vi "PlayFile.vi"(11 "Old Files":T1[](array[typedef])) -> ()   [LabVIEW 2022 SP3]
uses:
  Curtin1_Label.ctl
panel:
  in  "Save Convolve":bool
  in  "Convolve":bool
  in  "Save Button":bool
  in  "Play Button":bool
  in  "Instruments":u16(ring) items=["JacksonStrad H.AvR"]
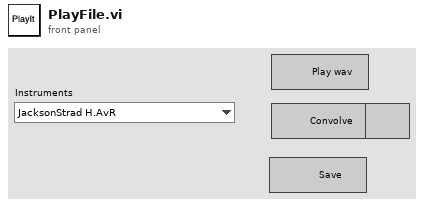
[diagram p1: front panel]
types:
  T1 = typedef "Curtin1_Label.ctl" = cluster{"Show?":bool, "Name":string, "Color":u32, "Path":path, "Show Notes":bool}
  T2 = typedef "PreferencesControl.ctl" = cluster{"Name of test":string, "Date":timestamp, "Location":string, "Template":string, "Soundcard":string, "resolution":u16, "Sampling rate":u16, "Ch1 Gain ":dbl, "Ch2 Gain":dbl, "Sample time (s)":dbl, "Pre-trigger (s)":dbl, "Hammer Threshold":dbl, "Positions":i16, "Taps/Position":i16, "Set Names":string, "Freq resolution":dbl, "Hammer cutoff":dbl, "Mic cutoff":dbl, "Double bounce ":dbl, "Hammer Cal":dbl, "dB Offset":dbl, "Accel Cal":dbl, "Vibrometer Cal":dbl, "Mic Cal":dbl, "Output":u16, "Voltage Cal":dbl, "Vibrometer Port":refnum<visa-resource-name>, "Range":u16, "High Pass":u16, "Bandwidth":u16, "X Range":cluster{"Minimum":dbl, "Maximum":dbl, "Increment":dbl, "Minor Increment":dbl, "Start":dbl}[], "Y Range":cluster{"Minimum":dbl, "Maximum":dbl, "Increment":dbl, "Minor Increment":dbl, "Start":dbl}[], "dB Spread":dbl, "Trigger":u16, "Ch_1":u8, "Ch_2":u8, "flip?":bool, "60Hz":bool, "Time offset":dbl, "Piezo Cal":dbl, "Default Notes":string}
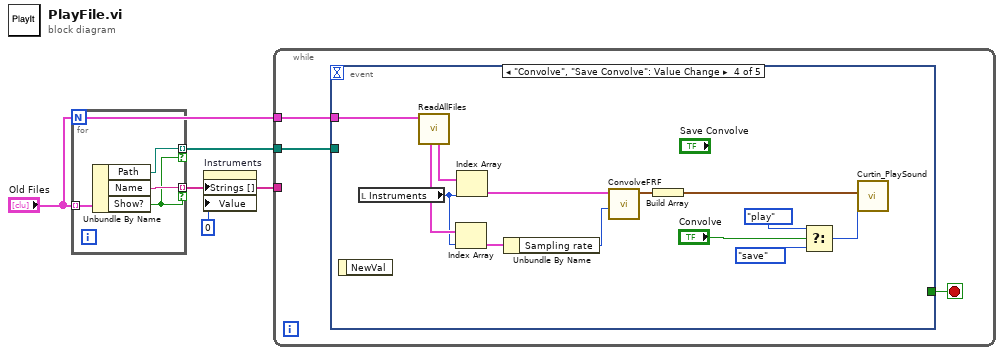
[diagram p0: block diagram]
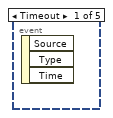
[diagram p2: hidden frame]
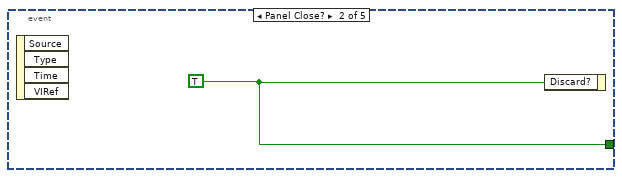
[diagram p3: hidden frame]
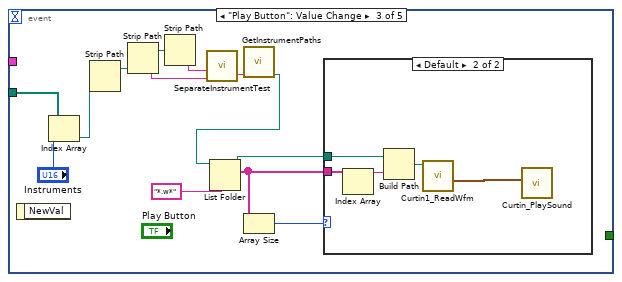
[diagram p4: hidden frame]
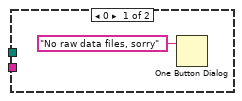
[diagram p5: hidden frame]
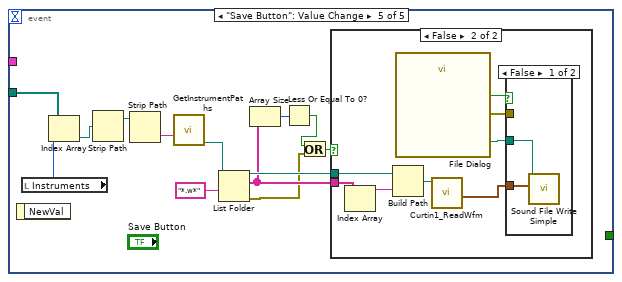
[diagram p6: hidden frame]
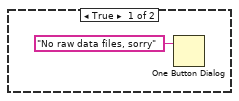
[diagram p7: hidden frame]
diagram:
  n1 = for {
    tunnel: "Old Files" -> [w8] mode=indexing
    tunnel: [w7] -> w3 mode=indexing if=w5
    tunnel: [w6] -> w2 mode=indexing if=w5
    n2 = Unbundle By Name(w8) -> ("Path"=w6:path, "Name"=w7:string, "Show?"=w5:bool)
  }
  n3 = property on="Instruments" class="Ring (strict)"("Strings []"=w3, "Value"=0) -> ()  [unwired: 2 in, 2 out]
  n4 = while {
    tunnel: w3 -> [_]
    tunnel: w2 -> [w10]
    tunnel: "Old Files" -> [w9]
    stop <- w11 stop-if-true
    n5 = event shown="[3] \"Convolve\", \"Save Convolve\": Value Change" {
      selector: _ -> [_ _ _ _ _]
      dyn-events: _ -> [_ _ _ _ _]
      timeout: _ -> [_ _ _ _ _]
      tunnel: [_ w12 _ _ _] -> w11
      tunnel: w10 -> [_ _ w21 _ w54]
      tunnel: w9 -> [_ _ _ w44 _]
      event Timeout {
        n6 = event-data() -> ()  [unwired: 1 in, 3 out]
      }
      event Panel Close? {
        w12 = TRUE ("Discard?")
        n7 = event-data() -> ()  [unwired: 1 in, 4 out]
        n8 = event-data("Discard?"=w12) -> ()  [unwired: 1 in, 1 out]
      }
      event "Play Button": Value Change {
        n9 = event-data() -> ()  [unwired: 1 in, 1 out]
        n10 = Index Array(array=w21, index="Instruments") -> (element=w13:path)
        n11 = Strip Path(path=w13) -> (stripped path=w20:path)  [unwired: 1 out]
        n12 = Strip Path(path=w20) -> (stripped path=w19:path, name=w17:string)
        n13 = Strip Path(path=w19) -> (name=w18:string)  [unwired: 1 out]
        n14 = call "SeparateInstrumentTest.vi"("test in"=w17, "Instrument in"=w18) -> ("Instrument -- test out"=w16:string)  [unwired: 5 in, 4 out]
        n15 = call "GetInstrumentPaths.vi"("Instrument"=w16) -> ("Path To Raw Folder"=w24:path)  [unwired: 6 in, 4 out]
        n16 = List Folder(path=w24, pattern="*.w*") -> (path out=w22:path, filenames=w15:string[])  [unwired: 2 in, 2 out]
        n17 = Array Size(array=w15) -> (size(s)=w14:i32)
        n18 = case shown="Default" w14 {
          tunnel: w22 -> [_ w30]
          tunnel: w15 -> [_ w29]
          frame 0 {
            n19 = One Button Dialog(message="No raw data files, sorry") -> ()  [unwired: 1 in, 1 out]
          }
          frame Default {
            n20 = Index Array(array=w29) -> (element=w31:string)  [unwired: 1 in]
            n21 = Build Path(base path=w30, name or relative path=w31) -> (appended path=w28:path)
            n22 = call "Curtin1_ReadWfm.vi"("appended path"=w28) -> ("all waveforms in record"=w27:waveform(dbl)[])  [unwired: 9 in, 1 out]
            n23 = call "Curtin_PlaySound.vi"("all waveforms"=w27) -> ()  [unwired: 10 in, 1 out]
          }
        }
      }
      event "Convolve", "Save Convolve": Value Change {
        n24 = event-data() -> ()  [unwired: 1 in, 1 out]
        n25 = local read "Instruments"() -> (w40:u16)
        n26 = call "ReadAllFiles.vi"("Files"=w44) -> ("data"=w43:cluster{"t0":dbl, "df":dbl, "Y":cdb[]}[], "Settings"=w41:T2[])  [unwired: 5 in, 4 out]
        n27 = Index Array(array=w41, index=w40) -> (element=w39:T2)
        n28 = Index Array(array=w43, index=w40) -> (element=w42:cluster{"t0":dbl, "df":dbl, "Y":cdb[]})
        n29 = Unbundle By Name(w39) -> ("Sampling rate"=w38:u16)
        n30 = call "ConvolveFRF.vi"("Sampling rate"=w38, "Complex FRF"=w42) -> ("Convolution"=w37:waveform(dbl))  [unwired: 7 in, 2 out]
        n31 = Build Array(w37) -> (w36:waveform(dbl)[])
        n32 = Select(t=enum16{"play", "save"}."play" ("Task"), s="Convolve", f=enum16{"play", "save"}."save" ("Task")) -> (s? t:f=w34:enum16{"play", "save"})
        n33 = call "Curtin_PlaySound.vi"("Task"=w34, "all waveforms"=w36) -> ()  [unwired: 9 in, 1 out]
      }
      event "Save Button": Value Change {
        n34 = event-data() -> ()  [unwired: 1 in, 1 out]
        n35 = local read "Instruments"() -> (w50:u16)
        n36 = Index Array(array=w54, index=w50) -> (element=w52:path)
        n37 = Strip Path(path=w52) -> (stripped path=w51:path)  [unwired: 1 out]
        n38 = Strip Path(path=w51) -> (name=w53:string)  [unwired: 1 out]
        n39 = call "GetInstrumentPaths.vi"("Instrument"=w53) -> ("Path To Raw Folder"=w57:path)  [unwired: 6 in, 4 out]
        n40 = List Folder(path=w57, pattern="*.w*") -> (path out=w55:path, filenames=w49:string[], error out=w46:errorcluster)  [unwired: 2 in, 1 out]
        n41 = Array Size(array=w49) -> (size(s)=w48:i32)
        n42 = Less Or Equal To 0?(x=w48) -> (x <= 0?=w47:bool)
        n43 = Or(x=w47, y=w46) -> (x .or. y?=w45:bool)
        n44 = case shown="False" w45 {
          tunnel: w49 -> [_ w66]
          tunnel: w55 -> [_ w64]
          frame True {
            n45 = One Button Dialog(message="No raw data files, sorry") -> ()  [unwired: 1 in, 1 out]
          }
          frame False {
            n46 = Index Array(array=w66) -> (element=w65:string)  [unwired: 1 in]
            n47 = Build Path(base path=w64, name or relative path=w65) -> (appended path=w63:path)
            n48 = call "File Dialog"() -> ("selected path"=w61:path, "cancelled"=w60:bool, "error out"=w59:errorcluster)  [unwired: 12 in, 1 out]
            n49 = call "Curtin1_ReadWfm.vi"("appended path"=w63) -> ("all waveforms in record"=w62:waveform(dbl)[])  [unwired: 9 in, 1 out]
            n50 = case shown="False" w60 {
              tunnel: w62 -> [w68 _]
              tunnel: w61 -> [w67 _]
              tunnel: w59 -> [_ _]
              frame False {
                n51 = call <vilib>:"Sound File Write Simple.vi"("data"=w68, "path"=w67) -> ()  [unwired: 8 in, 2 out]
              }
              frame True {
              }
            }
          }
        }
      }
    }
  }
